vi "STE.vi"(0 "System no.":i32=1 min=1 max=4 step=1, 2 "Axis to command":string, 3 "Step size":dbl format="%.6f", 4 "No.of digits":i16=4, 5 "error in":errorcluster, 6 "Delay":i32) -> (19 "error out":errorcluster)   [LabVIEW 2020]
doc: "Performs a single step-move from the current position with specified step size (amplitude). If supported, Delay defines the number of servo loops between position recording (GCS 2.0: Delay must be 0). Controller saves a definite number of position values, which can be read out with STE?.vi (GCS 1.0) or DRR? (GCS 2.0). No. of digits is the number of digits after the decimal point in the step size values that will be sent. For an impulse-move, see IMP.vi.\n\nAnalog: Delay = 0. Use DRR?.vi or DRR? and display data.vi to read position values back.\n\nC-843: Controller saves up to 32,640 position values for all 4 channels in sum. Delay = 0. Use STE?.vi to read position values back.\n\nC-843.PM: Controller saves up to 32,640 position values for all 4 channels in sum. Delay = 0. Use STE?.vi to read position values back.\n\nC-848: Controller saves 1024 position values. Use STE?.vi to read position values back.\n\nC-865: Controller saves up to 32,640 position values. Delay = 0. Use STE?.vi to read position values back.\n\nC-866: Controller saves up to 32,256 position values. STE will overwrite DRC settings of Rec. table 1 to record actual position values. Use DRC to define additional record options for Rec. table no. 2 to 4. Record table rate is reset to 1 by STE. Use STE?.vi to read position values back or DRR? to read all Rec. tables back. You can also use MVR in combination with DRC to record values of a step motion. Use DRR? to read values back then.\n\nC-867: Controller saves up to 8192 position values.\nMotion commands like STE are not allowed when the joystick is active for the axis. Use DRC to define record options. Use DRR?.vi or DRR? and display data.vi to read recorded values back. You can also use MVR in combination with DRC to record values of a step motion.\n\nC-877: See user manual for available record options, number of data recorder tables and points per table. Use DRC to define record options. Use DRR?.vi or DRR? and display data.vi to read recorded values back. You can also use MVR in combination with DRC to record values of a step motion.\n\nC-880: Controller saves 1024 position values. Use STE?.vi to read position values back.\n\nC-884: Controller saves 8192 position values. Motion commands like STE are not allowed when control via a Human Interface Device (HID) is active for the axis of the controller. Use DRC to define record options. Use DRR?.vi or DRR? and display data.vi to read recorded values back. You can also use MVR in combination with DRC to record values of a step motion.\n\nC-891: See Controller user manual for details. Use DRC to define record options. Use DRR?.vi or DRR? and display data.vi to read recorded values back. You can also use MVR in combination with DRC to record values of a step motion.\n\nE-517, E-518: Controller saves up to 8,192 position values. Use DRR?.vi or DRR?and display data.vi to read recorded values back. The number of servocycles used for data recording depends on the setting made with RTR.\nMotion commands like STE are not allowed when the controller is in OFFLINEmode or when the wave generator output is active. When a macro is running on the controller, STE will be executed not until the macro is finished or stopped. See\"Control Value Generation\" and \"Control Modes\" in the controller user manual for details.\n\nC-413, E-709: Controller saves up to 4096 position values. Use DRR?.vi or DRR? and display data.vi to read recorded values back. The number of servo cycles used for data recording depends on the setting made with RTR. Motion commands are not allowed when the wave generator is active or the analog input is used for target generation.\n\nE-710: Controller saves 32256 position values. Delay = 0. \"Table Rate\" parameter, set with SPA.vi, is used as sampling interval instead of Delay. Caution: \"Table Rate\" parameter influences wave generator also, not only STE. Use STE?.vi to read position values back.\n\nE-712: Controller saves up to 262,144 position values. Use DRR?.vi or DRR? and display data.vi to read recorded values back. The number of servo cycles used for data recording depends on the setting made with RTR. Motion commands are not allowed when a wave generator is active or the analog input is used for target generation.\n\nE-725, E-727: Controller saves up to 262,144 position values. Use DRR?.vi or DRR? and display data.vi to read recorded values back. The number of servo cycles used for data recording depends on the setting made with RTR. Motion commands are not allowed when a wave generator is active or the analog input is used for target generation.\n\nE-753: Controller saves up to 65,536 position values. Use DRR?.vi or DRR? and display data.vi to read recorded values back. The number of servo cycles used for data recording depends on the setting made with RTR. Motion commands are not allowed when the wave generator is active or the analog input is used for target generation.\n\nE-754: Controller saves up to 1,048,576 position values. Use DRR?.vi or DRR? and display data.vi to read recorded values back. The number of servo cycles used for data recording depends on the setting made with RTR. Motion commands are not allowed when the wave generator is active or the analog input is used for target generation.\n\nE-755: Delay = 0. Controller saves 4096 position values. Use DRR?.vi or DRR? and display data.vi to read recorded values back.\n\nE-761: Controller saves 8192 position values. Delay = 0. The number of servo cycles used for data recording depends on the setting made with RTR.vi. Use DRR?.vi or STE?.vi to read position values back.\n\nE-861: Step response measurements provide meaningful results only in closed-loop operation. Controller saves up to 1,024 position values.\nMotion commands like STE are not allowed when the joystick is active for the axis. Use DRC to define record options. Use DRR?.vi or DRR? and display data.vi to read recorded values back. You can also use MVR in combination with DRC to record values of a step motion. \n\nE-871, E-873, E-874: Controller saves up to 1024 position values.\nMotion commands like STE are not allowed when the joystick is active for the axis. Use DRC to define record options. Use DRR?.vi or DRR? and display data.vi to read recorded values back. You can also use MVR in combination with DRC to record values of a step motion.\n\nC-887, F-206, M-8X0: Controller saves 1,024 position values (number can be changed by setting the appropriate parameter value, see user manual). Use DRR?.vi or DRR? and display data.vi to read recorded values back. Only for GCS syntax version = GCS 2.0 or higher (check with CSV?.vi. If CSV?.vi is not supported, syntax version is GCS 1.0).\n\nMercury_GCS: Controller saves up to 1,024 position values. Motion commands like STE are not allowed when the joystick is active for the axis. Use DRC to define record options. Use DRR?.vi or DRR? and display data.vi to read recorded values back. You can also use MVR in combination with DRC to record values of a step motion."
panel:
  # "Performs a single step-move from the current \nposition with specified step size (amplitude). If supported, \n\"Delay\" defines the number of servo loops between position \nrecording. Controller saves a definite number of position values, \nwhich can be read out with STE?.vi (GCS 1.0) or DRR?.vi (GCS 2.0)."
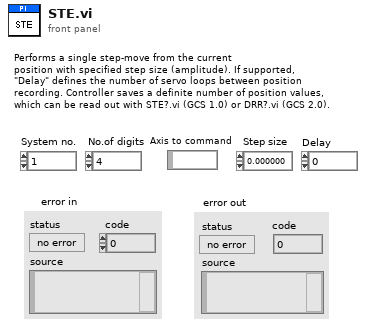
[diagram p1: front panel]
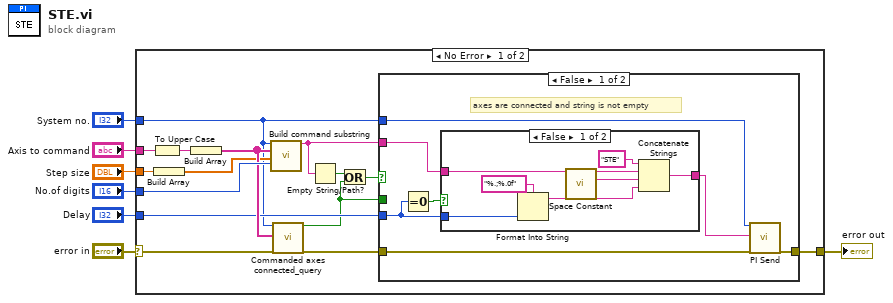
[diagram p0: block diagram]
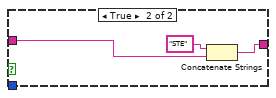
[diagram p2: hidden frame]
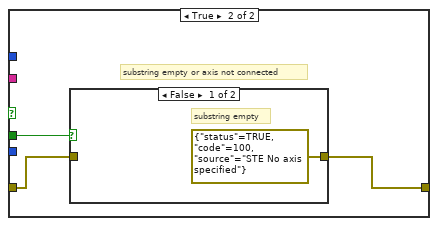
[diagram p3: hidden frame]
diagram:
  n1 = case shown="No Error" "error in" {
    selector: "error in" -> [w8 w45]
    tunnel: [w22 w45] -> w7
    tunnel: "No.of digits" -> [w21 _]
    tunnel: "System no." -> [w12 _]
    tunnel: "Step size" -> [w17 _]
    tunnel: "Axis to command" -> [w15 _]
    tunnel: "Delay" -> [w13 _]
    frame No Error {
      n2 = To Upper Case(1:w15) -> (0:w14:string)
      n3 = Build Array(w17) -> (w16:dbl[])
      n4 = Build Array(w14) -> (w18:string[])
      n5 = call "Build command substring.vi"("System no."=w12, "Affected axes"=w18, "Parameters"=w16, "No. of digits"=w21) -> ("Command substring"=w9:string)  [unwired: 3 in, 12 out]
      n6 = call "Commanded axes connected_query.vi"("System no."=w12, "Commanded axes"=w18, "error in"=w8) -> ("Controller error"=w11:bool, "error out"=w20:errorcluster)  [unwired: 1 in, 14 out]
      n7 = Empty String/Path?(string/path=w9) -> (empty?=w10:bool)
      n8 = Or(x=w10, y=w11) -> (x .or. y?=w19:bool)
      n9 = case shown="False" w19 {
        tunnel: w9 -> [w29 _]
        tunnel: [w26 w42] -> w22
        tunnel: w20 -> [w27 w40]
        tunnel: w11 -> [_ w41]
        tunnel: w12 -> [w25 _]
        tunnel: w13 -> [w24 _]
        frame False {
          # "axes are connected and string is not empty"
          n10 = Equal To 0?(x=w24) -> (x = 0?=w23:bool)
          n11 = case shown="False" w23 {
            tunnel: w29 -> [w35 w38]
            tunnel: [w34 w37] -> w28
            tunnel: w24 -> [w32 _]
            frame False {
              n12 = Format Into String(format string="%.;%.0f" ("Format String"), w32) -> (resulting string=w30:string)  [unwired: 2 in, 1 out]
              n13 = call "Space Constant.vi"() -> ("String"=w31:string)
              n14 = Concatenate Strings("STE", w35, w31, w30) -> (w34:string)
            }
            frame True {
              n15 = Concatenate Strings("STE", w38) -> (w37:string)
            }
          }
          n16 = call "PI Send.vi"("System no."=w25, "String to send"=w28, "error in"=w27) -> ("error out"=w26:errorcluster)  [unwired: 3 in, 13 out]
        }
        frame True {
          # "substring empty or axis not connected"
          n17 = case shown="False" w41 {
            tunnel: [errorcluster {"status"=TRUE, "code"=100, "source"="STE No axis specified"} ("error out") w44] -> w42
            tunnel: w40 -> [_ w44]
            frame False {
              # "substring empty"
            }
            frame True {
              # "commanded axis not connected"
            }
          }
        }
      }
    }
    frame Error {
    }
  }
  "error out" <- w7
